vi "log_watcher.vi"() -> ()   [LabVIEW 2012]
uses:
  log_event.ctl
  <vilib>/Platform/TimedLoop/XDataNode/timing_clust.ctl
  <vilib>/Platform/TimedLoop/XDataNode/nitl_modes.ctl
  <vilib>/Platform/TimedLoop/XDataNode/wakeup.ctl
  <vilib>/Platform/TimedLoop/XDataNode/XDataNode.xnode
  <vilib>/Platform/TimedLoop/XDataNode/XDNodeRunTimeDep.lvlib
panel:
  in  "Log size":i32=100
  in  "Save":bool caption="Clear"
  in  "Log file":path
  out "Events":i32
  in  "stop":bool
  in  "Clear":bool
  out "Event log":T1[](array[typedef]) {"Timestamp" format="%<%.3X>T"}
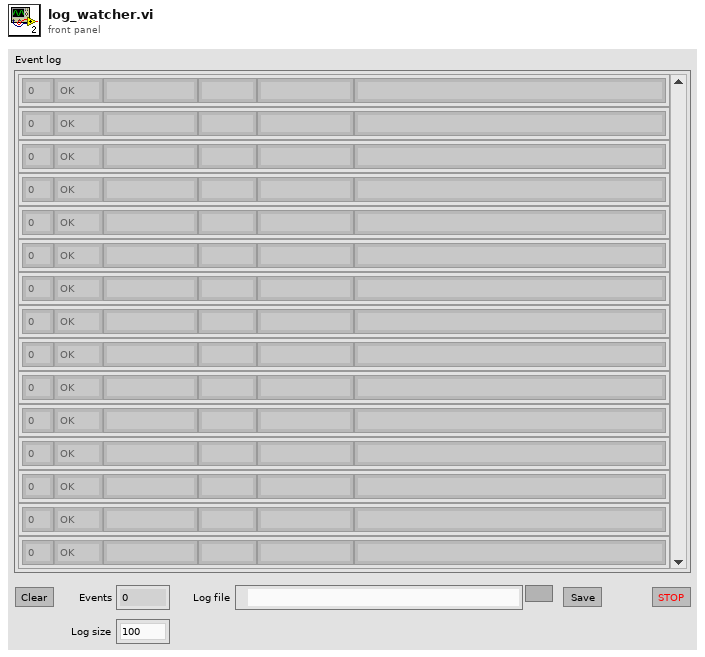
[diagram p1: front panel]
types:
  T1 = typedef "log_event.ctl" = cluster{"Facility ID":i32, "Severity":enum16{"OK", "Debug", "Warn", "Error"}, "Timestamp":timestamp, "Facility":string, "State":string, "Message":string}
  T2 = typedef "XDNodeRunTimeDep.lvlib/timing_clust.ctl" = cluster{"Expected End [f-1]":u64, "Actual End [f-1]":u64, "Finished Late? [f-1]":bool, "Expected End [i-1]":u64, "Actual End [i-1]":u64, "Finished Late? [i-1]":bool, "Expected Start [i]":u64, "Actual Start [i]":u64, "Expected Start [f]":u64, "Actual Start [f]":u64, "Source Name":string, "Structure Name":string, "Period":i64, "Deadline":i64, "Offset":i64, "Start":i64, "Priority":i32, "Timeout":i32, "Mode":T3, "Wakeup Reason":T4, "Error":errorcluster, "Source Type":string, "Secondary Source Type":string, "Global End Time":u64, "Global Start Time":u64, "Frame Duration":u64, "Iteration Duration":u64, "Assigned CPU":i32, "I/O Scan Engine Mode":u32}
  T3 = typedef "XDNodeRunTimeDep.lvlib/nitl_modes.ctl" = enum32{"No Change", "Process missed periods, maintain original phase", "Discard missed periods, maintain original phase", "Process missed periods, ignore original phase", "Discard missed periods, ignore original phase"}
  T4 = typedef "XDNodeRunTimeDep.lvlib/wakeup.ctl" = enum32{"Normal", "Aborted", "Asynchronous wakeup", "Timing source error", "Timed loop error", "Timeout"}
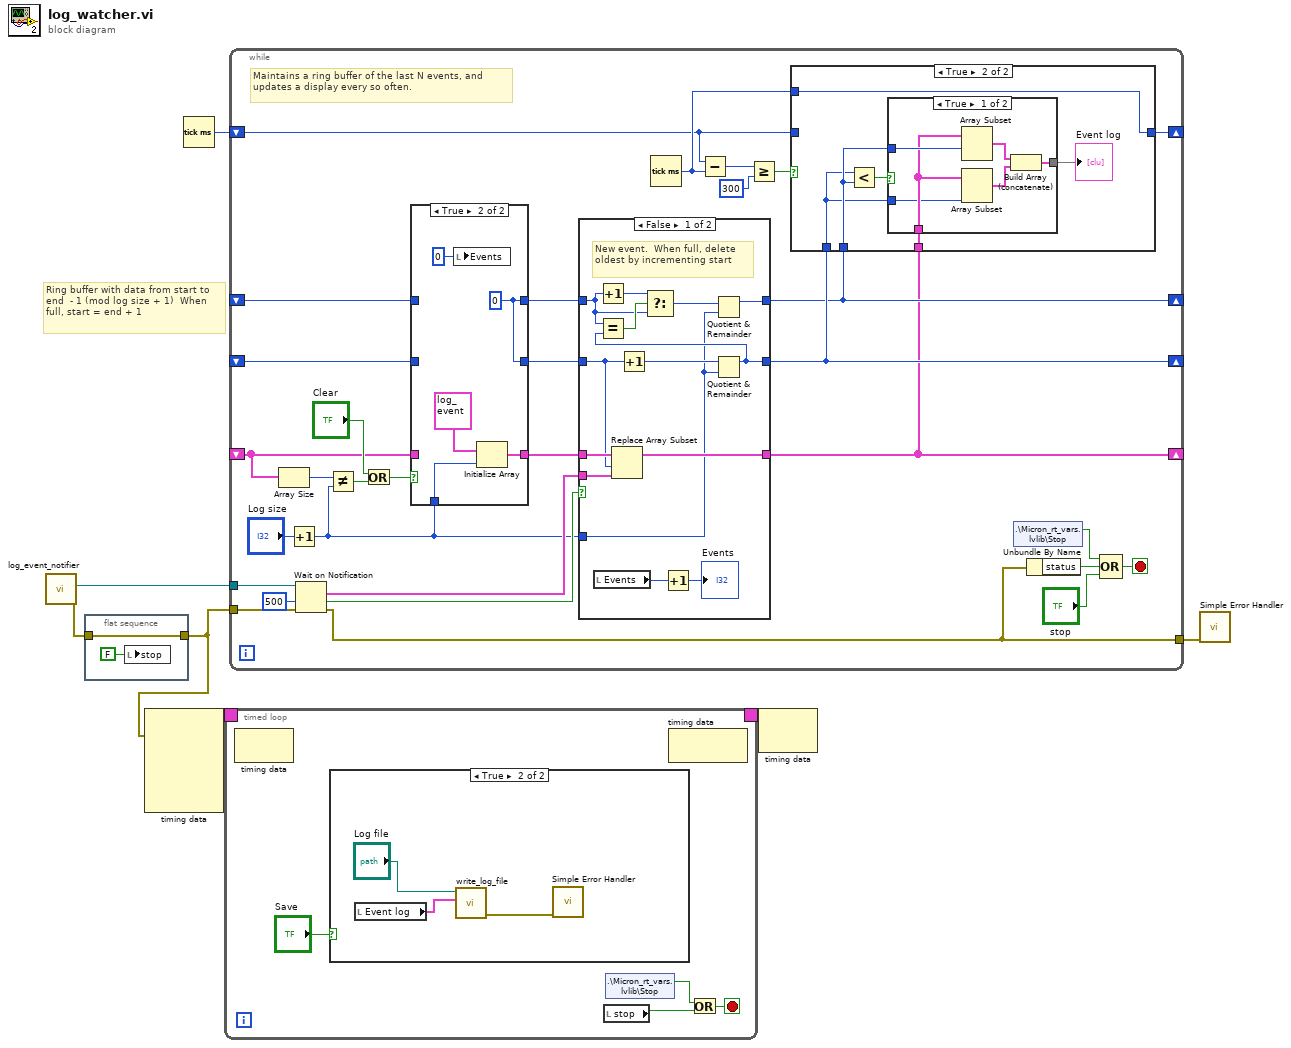
[diagram p0: block diagram]
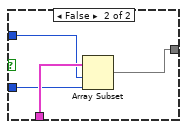
[diagram p4: hidden frame]
diagram:
  # "Ring buffer with data from start to  end  - 1 (mod log size + 1)  When full, start = end + 1"
  n1 = call "log_event_notifier.vi"() -> ("error out"=w4:errorcluster, "Log event notifier"=w7:refnum<notifier>)  [unwired: 10 in]
  n2 = flat-sequence {
    tunnel: w4 -> [w8]
    tunnel: [w8] -> w3
    frame #0 {
      n3 = local write "stop"(FALSE ("stop")) -> ()
    }
  }
  n4 = node-c288(w3) -> (w6:T2)  [unwired: 4 in]
  n5 = Tick Count (ms)() -> (millisecond timer value=w2:u32)
  n6 = timed-loop {
    timing: w6 -> [_]
    timing-out: [_] -> w5
    stop <- w10 stop-if-true
    n7 = node-c288() -> ()  [unwired: 1 in, 1 out]
    n8 = case shown="True" "Save" {
      frame False {
      }
      frame True {
        n9 = local read "Event log"() -> (w15:T1[])
        n10 = call "write_log_file.vi"("Event log"=w15, "Log file"="Log file") -> ("error out"=w14:errorcluster)  [unwired: 9 in]
        n11 = call <vilib>:"Simple Error Handler.vi"("error in (no error)"=w14) -> ()  [unwired: 4 in, 5 out]
      }
    }
    n12 = local read "stop"() -> (w11:bool)
    n13 = shared-variable ".\\Micron_rt_vars.lvlib\\Stop"() -> (w12:bool)  [unwired: 1 in, 1 out]
    n14 = node-c288() -> ()  [unwired: 1 in, 1 out]
    n15 = Or(x=w12, y=w11) -> (x .or. y?=w10:bool)
  }
  n16 = while {
    tunnel: w7 -> [w49]
    tunnel: w3 -> [w48]
    tunnel: [w40] -> w1
    shift-right: [w22] -> _
    shift-left: _ -> [w36]
    shift-right: [w24] -> _
    shift-left: _ -> [w34]
    shift-right: [w23] -> _
    shift-left: _ -> [w33]
    shift-right: [w25] -> _
    shift-left: w2 -> [w21]
    stop <- w42 stop-if-true
    # "Maintains a ring buffer of the last N events, and updates a display every so often."
    n17 = Array Size(array=w36) -> (size(s)=w39:i32)
    n18 = Increment(x="Log size") -> (x+1=w19:i32)
    n19 = Wait on Notification(notifier=w49, timeout in ms (-1)=500, error in (no error)=w48) -> (notification=w45:T1, timed out?=w46:bool, error out=w40:errorcluster)  [unwired: 1 in, 1 out]
    n20 = Not Equal?(x=w39, y=w19) -> (x != y?=w38:bool)
    n21 = Or(x="Clear", y=w38) -> (x .or. y?=w35:bool)
    n22 = case shown="True" w35 {
      tunnel: w36 -> [w67 _]
      tunnel: w19 -> [_ w70]
      tunnel: [w67 w73] -> w32
      tunnel: w34 -> [w68 _]
      tunnel: w33 -> [w69 _]
      tunnel: [w69 w72] -> w30
      tunnel: [w68 w72] -> w31
      frame False {
      }
      frame True {
        w72 = 0 ("Log size")
        n23 = local write "Events"(0 ("Events")) -> ()
        n24 = Initialize Array(T1 {"Facility ID"=0, "Severity"=enum."OK", "Timestamp"=timestamp(0 s since 1904-01-01), "Facility"="", "State"="", "Message"=""} ("Log event"), w70) -> (w73:T1[])
      }
    }
    n25 = case shown="False" w46 {
      tunnel: w45 -> [w87 _]
      tunnel: w32 -> [w88 w91]
      tunnel: [w83 w91] -> w22
      tunnel: w31 -> [w86 w90]
      tunnel: w30 -> [w80 w89]
      tunnel: [w78 w90] -> w24
      tunnel: [w77 w89] -> w23
      tunnel: w19 -> [w76 _]
      frame False {
        # "New event.  When full, delete oldest by incrementing start"
        n26 = local read "Events"() -> (w82:i32)
        n27 = Increment(x=w80) -> (x+1=w84:i32)
        n28 = Replace Array Subset(array=w88, new element=w87, index=w86) -> (w83:T1[])
        n29 = Increment(x=w86) -> (x+1=w79:i32)
        n30 = Increment(x=w82) -> (x+1=→"Events":i32)
        n31 = Quotient & Remainder(x=w79, y=w76) -> (x-y*floor(x/y)=w78:i32)  [unwired: 1 out]
        n32 = Equal?(x=w80, y=w78) -> (x = y?=w85:bool)
        n33 = Select(t=w84, s=w85, f=w80) -> (s? t:f=w75:i32)
        n34 = Quotient & Remainder(x=w75, y=w76) -> (x-y*floor(x/y)=w77:i32)  [unwired: 1 out]
      }
      frame True {
      }
    }
    n35 = Tick Count (ms)() -> (millisecond timer value=w26:u32)
    n36 = Subtract(x=w21, y=w26) -> (x-y=w29:u32)
    n37 = Greater Or Equal?(x=w29, y=u32 300) -> (x >= y?=w27:bool)
    n38 = case shown="True" w27 {
      tunnel: w26 -> [_ w56]
      tunnel: [w50 w56] -> w25
      tunnel: w24 -> [_ w52]
      tunnel: w23 -> [_ w53]
      tunnel: w22 -> [_ w54]
      tunnel: w21 -> [w50 _]
      frame False {
      }
      frame True {
        n39 = Less?(x=w52, y=w53) -> (x < y?=w55:bool)
        n40 = case shown="True" w55 {
          tunnel: w54 -> [w61 w66]
          tunnel: w53 -> [w62 w65]
          tunnel: w52 -> [w57 w63]
          tunnel: [w58 w64] -> w51
          frame True {
            n41 = Array Subset(array=w61, index=w62) -> (w60:T1[])  [unwired: 1 in]
            n42 = Array Subset(array=w61, length=w57) -> (w59:T1[])  [unwired: 1 in]
            n43 = Build Array (concatenate)(w60, w59) -> (w58:T1[])
          }
          frame False {
            n44 = Array Subset(array=w66, index=w65, length=w63) -> (w64:T1[])
          }
        }
        "Event log" <- w51
      }
    }
    n45 = shared-variable ".\\Micron_rt_vars.lvlib\\Stop"() -> (w44:bool)  [unwired: 1 in, 1 out]
    n46 = Unbundle By Name(w40) -> ("status"=w43:bool)
    n47 = Compound Arithmetic op=OR(w44, w43, "stop") -> (w42:bool)
  }
  n48 = node-c288(w5) -> ()  [unwired: 1 out]
  n49 = call <vilib>:"Simple Error Handler.vi"("error in (no error)"=w1) -> ()  [unwired: 4 in, 5 out]
